vi "Config Audio UI.vi"() -> ()   [LabVIEW 2013]
panel:
  in  "Speakers":u32(ring) items=["Speakers / HP (IDT High Definition Audio CODEC)", "Headphones (RTC) (IDT High Definition Audio CODEC)"]
  in  "Microphone":u32(ring) items=["Integrated Microphone Array (IDT High Definition Audio CODEC)", "Microphone (IDT High Definition Audio CODEC)", "Rec. Playback (IDT High Definition Audio CODEC)", "Line In (IDT High Definition Audio CODEC)"]
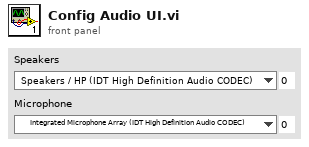
[diagram p1: front panel]
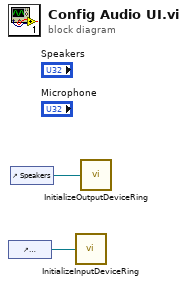
[diagram p0: block diagram]
diagram:
  n1 = control-ref of="Microphone"() -> (w2:refnum<vi>)
  n2 = control-ref of="Speakers"() -> (w1:refnum<vi>)
  n3 = call <vilib>:"InitializeInputDeviceRing.vi"("Device Refnum"=w2) -> ()  [unwired: 14 in, 1 out]
  n4 = call <vilib>:"InitializeOutputDeviceRing.vi"("Device Refnum"=w1) -> ()  [unwired: 14 in, 1 out]
